vi "Get SubpanelVI Info.vi"(8 "error in (no error)":errorcluster, 11 "MotionSystem Configuration in":refnum<class "MotionSystem Configuration.lvclass">) -> (0 "error out":errorcluster, 1 "Array of Subpanel VI data":T1[](array[typedef]), 2 "Array of Category string":string[](array[string]), 3 "MotionSystem Configuration out":refnum<class "MotionSystem Configuration.lvclass">)   [LabVIEW 2016, in "MotionSystem.lvlib" / "MotionSystem Configuration.lvclass"]
uses:
  <userlib>/Common Components/Hardware/Abstract System/MotionSystem/MotionSystem Config/MotionSystem Configuration.lvclass
  <userlib>/Configuration Dialog Actor/Methods/Data Retrieved by Lookup Table.ctl
  <userlib>/Configuration Dialog Actor/Configuration.lvclass
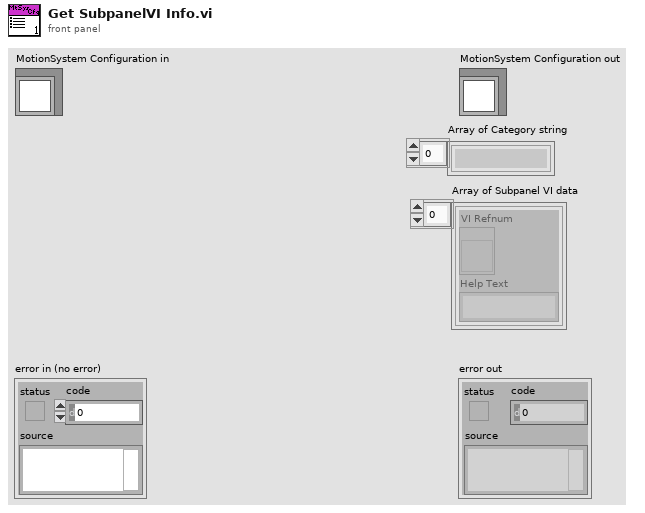
[diagram p1: front panel]
types:
  T1 = typedef "Configuration.lvlib/Configuration.lvclass/Data Retrieved by Lookup Table.ctl" = cluster{"VI Refnum":refnum<vi>, "Help Text":string}
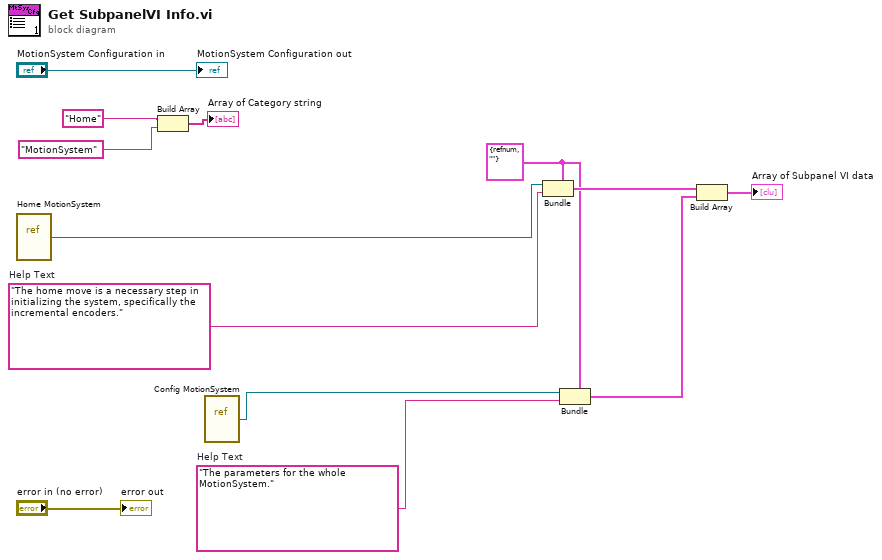
[diagram p0: block diagram]
diagram:
  w1 = "The parameters for the whole MotionSystem."  # Help Text
  w4 = T1 {"VI Refnum"=refnum, "Help Text"=""} ("output cluster")
  w10 = "The home move is a necessary step in initializing the system, specifically the incremental encoders."  # Help Text
  n1 = vi-ref <userlib>:"Home MotionSystem.vi"() -> (w11:refnum<vi>)
  n2 = Build Array("Home" ("Category string"), "MotionSystem" ("Category string")) -> (→"Array of Category string":string[])
  n3 = vi-ref <userlib>:"Config MotionSystem.vi"() -> (w2:refnum<vi>)
  n4 = Bundle(cluster=w4, "VI Refnum"=w11, "Help Text"=w10) -> (w7:T1)
  n5 = Bundle(cluster=w4, "VI Refnum"=w2, "Help Text"=w1) -> (w3:T1)
  n6 = Build Array(w7, w3) -> (→"Array of Subpanel VI data":T1[])
  "error out" <- "error in (no error)"
  "MotionSystem Configuration out" <- "MotionSystem Configuration in"
